vi "niHWS Close File.vi"(8 "error in (no error)":errorcluster, 11 "file handle":u32) -> (0 "error out":errorcluster)   [LabVIEW 2013]
doc: "Closes the HWS file specified by <B>file handle</B>."
uses:
  nihwsu.dll
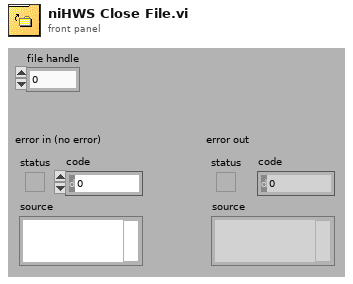
[diagram p1: front panel]
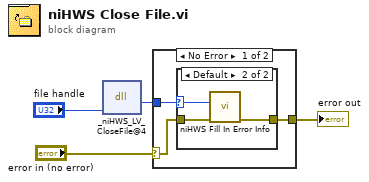
[diagram p0: block diagram]
diagram:
  n1 = dll-call lib="nihwsu.dll" fn="_niHWS_LV_CloseFile@4"("fileHandle"="file handle") -> (w1:i32)  [unwired: 4 in, 2 out]
  n2 = case shown="No Error" "error in (no error)" {
    selector: "error in (no error)" -> [w6 w12]
    tunnel: [w7 w12] -> w3
    tunnel: w1 -> [w5 _]
    frame No Error {
      n3 = case shown="Default" w5 {
        selector: w5 -> [_ w9]
        tunnel: [w8 w10] -> w7
        tunnel: w6 -> [w8 w11]
        frame 0 {
        }
        frame Default {
          n4 = call "niHWS Fill In Error Info.vi"("error in (no error)"=w11, "status code"=w9) -> ("error out"=w10:errorcluster)  [unwired: 9 in]
        }
      }
    }
    frame Error {
    }
  }
  "error out" <- w3
